vi "test GUI Interlock Tester-Power Off.vi"(8 "error in (no error)":errorcluster, 11 "TestCase in":refnum<class "GUI Interlock Tester.lvclass">) -> (0 "error out":errorcluster, 3 "TestCase out":refnum<class "GUI Interlock Tester.lvclass">)   [LabVIEW 2018, in "GUI Interlock Tester.lvclass"]
uses:
  GUI Interlock Tester.lvclass
  GUI Interlock Tester.lvclass/GUI Interlock Tester.ctl
  Libraries/Device Under Test_Cloneable_DQMH/Device Under Test_Cloneable_DQMH.lvlib
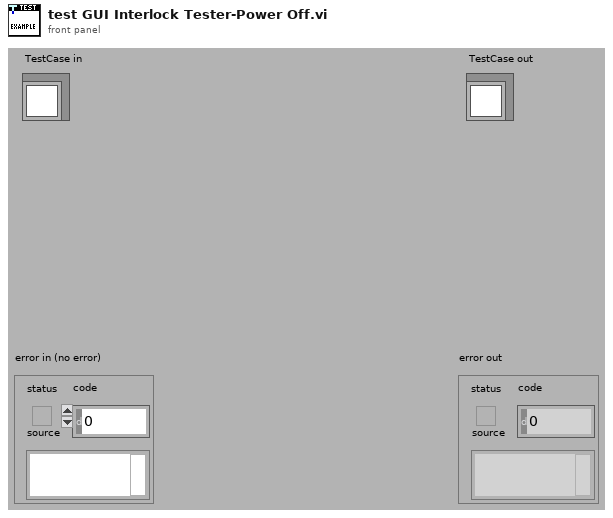
[diagram p1: front panel]
types:
  T1 = enum8{"Enabled", "Disabled", "Disabled and Grayed Out"}
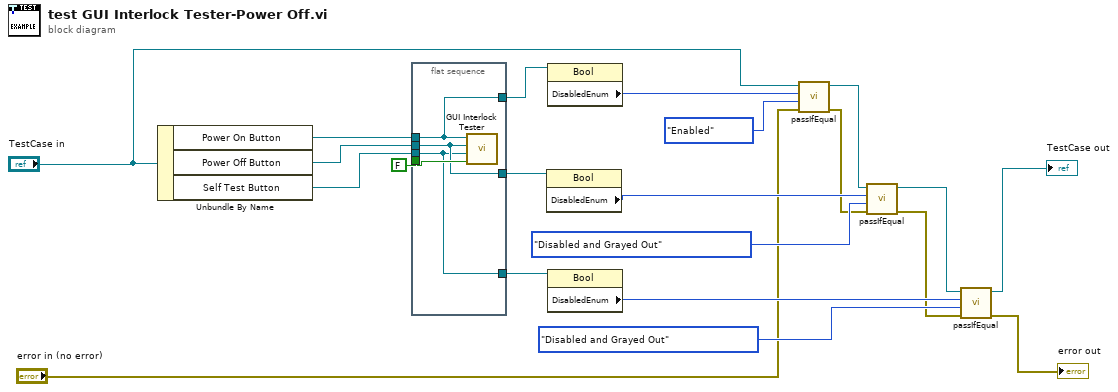
[diagram p0: block diagram]
diagram:
  n1 = Unbundle By Name("TestCase in") -> ("Power On Button"=w21:refnum<vi>, "Power Off Button"=w20:refnum<vi>, "Self Test Button"=w19:refnum<vi>)
  n2 = flat-sequence {
    tunnel: w21 -> [w24]
    tunnel: w20 -> [w23]
    tunnel: w19 -> [w22]
    tunnel: FALSE ("Power State") -> [w25]
    tunnel: [w24] -> w17
    tunnel: [w23] -> w16
    tunnel: [w22] -> w15
    frame #0 {
      n3 = call "GUI Interlock Tester.vi"("Power State"=w25, "Self Test Button"=w22, "Power Off Button"=w23, "Power On Button"=w24) -> ()  [unwired: 8 in]
    }
  }
  n4 = property class="Bool"(reference=w16) -> ("DisabledEnum"=w12:T1)  [unwired: 1 in, 2 out]
  n5 = property class="Bool"(reference=w17) -> ("DisabledEnum"=w14:T1)  [unwired: 1 in, 2 out]
  n6 = property class="Bool"(reference=w15) -> ("DisabledEnum"=w9:T1)  [unwired: 1 in, 2 out]
  n7 = call-dynamic "passIfEqual.vi"("error in (no error)"="error in (no error)", "y"=T1."Enabled" ("Disabled"), "x"=w14, "TestCase in"="TestCase in") -> ("error out"=w6:errorcluster, "TestCase out"=w10:refnum<class "GUI Interlock Tester.lvclass">)  [unwired: 6 in]
  n8 = call-dynamic "passIfEqual.vi"("error in (no error)"=w6, "y"=T1."Disabled and Grayed Out" ("Disabled"), "x"=w12, "TestCase in"=w10) -> ("error out"=w5:errorcluster, "TestCase out"=w7:refnum<class "GUI Interlock Tester.lvclass">)  [unwired: 6 in]
  n9 = call-dynamic "passIfEqual.vi"("error in (no error)"=w5, "y"=T1."Disabled and Grayed Out" ("Disabled"), "x"=w9, "TestCase in"=w7) -> ("error out"=→"error out":errorcluster, "TestCase out"=→"TestCase out":refnum<class "GUI Interlock Tester.lvclass">)  [unwired: 6 in]
